vi "CreatePath_WriteFGV_Example.vi"   [LabVIEW 2019]
panel:
  # "Create Trajectory and Write to Functional Global Variable"
  # "See block diagram"
types:
  T1 = typedef "PathPlanner24.lvlib/PathPlannerTrajectory.ctl" = cluster{"States":T2[]}
  T2 = typedef "PathPlanner24.lvlib/PathPlannerTrajectoryState.ctl" = cluster{"TimeSeconds":dbl, "VelocityMPS":dbl, "AccerationMpsSq":dbl, "HeadingAngularVelRadPerSec":dbl, "PositionMeters":T3, "Heading":T4, "TargetHolonomicRotation":T4, "CurvatureRadPerMeter":dbl, "PathPlannerConstraints":T5, "DeltaPos":dbl}
  T3 = typedef "Trajectory_Library.lvlib/TRANSLATION2D.ctl" = cluster{"X":dbl, "Y":dbl}
  T4 = typedef "Trajectory_Library.lvlib/ROTATION2D.ctl" = cluster{"VALUE":dbl, "COS":dbl, "SIN":dbl}
  T5 = typedef "PathPlanner24.lvlib/PathPlannerPathConstraints.ctl" = cluster{"MaxVelocityMps;":dbl, "MaxAccelerationMpsSq;":dbl, "MaxAngularVelRadPsEc;":dbl, "MaxAngularAccRadPSecSq":dbl, "Exists":bool}
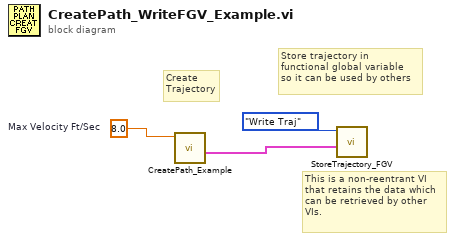
[diagram p0: block diagram]
diagram:
  w2 = 8.0  # Max Velocity Ft/Sec
  # "This is a non-reentrant VI\nthat retains the data which\ncan be retrieved by other\nVIs."
  # "Create\nTrajectory"
  # "Store trajectory in\nfunctional global variable\nso it can be used by others"
  n1 = call "CreatePath_Example.vi"("Max Velocity M/S"=w2) -> ("PathPlannerTrajectory"=w3:T1)  [unwired: 8 in, 2 out]
  n2 = call "StoreTrajectory_FGV.vi"("inTRAJECTORY"=w3, "Command"=enum16{"Sample", "Read Traj", "Write Traj"}."Write Traj") -> ()  [unwired: 8 in, 2 out]
